vi "Define Units.vi"(8 "error in":errorcluster, 11 "AI Arms channel in":refnum<class "AI Arms Channel.lvclass">) -> (0 "error out":errorcluster, 3 "AI Arms channel out":refnum<class "AI Arms Channel.lvclass">)   [LabVIEW 2020, in "Scan Engine Scripting.lvlib" / "AI Arms Channel.lvclass"]
uses:
  AI Arms Channel.lvclass
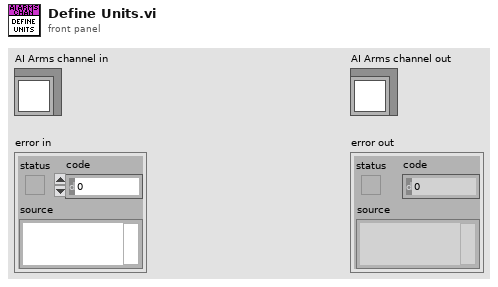
[diagram p1: front panel]
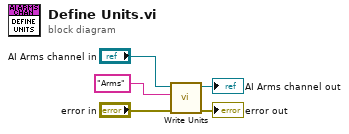
[diagram p0: block diagram]
diagram:
  n1 = call-dynamic "Write Units.vi"("error in"="error in", "units"="Arms", "channel in"="AI Arms channel in") -> ("error out"=→"error out":errorcluster, "channel out"=→"AI Arms channel out":refnum<class "AI Arms Channel.lvclass">)  [unwired: 7 in]
